vi "Splash Screen Main.vi"() -> ()   [LabVIEW 2020]
uses:
  <vilib>/LAVA/UI Tools/Fading/SetTransparency(U8)__lava_lib_ui_tools.vi
  <vilib>/LAVA/UI Tools/Fading/_Fade In(I32)__lava_lib_ui_tools.vi
  <vilib>/LAVA/UI Tools/Fading/_Fade Out(I32)__lava_lib_ui_tools.vi
panel:
  out "Logo":picture
  out "Status Indicator":string
  out "Splash Indicator Cluster":T1
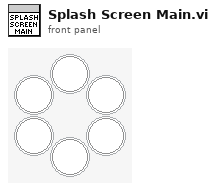
[diagram p1: front panel]
types:
  T1 = cluster{"Indicator 1":bool, "Indicator 2":bool, "Indicator 3":bool, "Indicator 4":bool, "Indicator 5":bool, "Indicator 6":bool}
  T2 = enum32{"Invalid", "Standard", "Closed", "Hidden", "Minimized", "Maximized"}
  T3 = cluster{"Indicator 6":bool, "Indicator 5":bool, "Indicator 3":bool, "Indicator 4":bool, "Indicator 2":bool, "Indicator 1":bool}
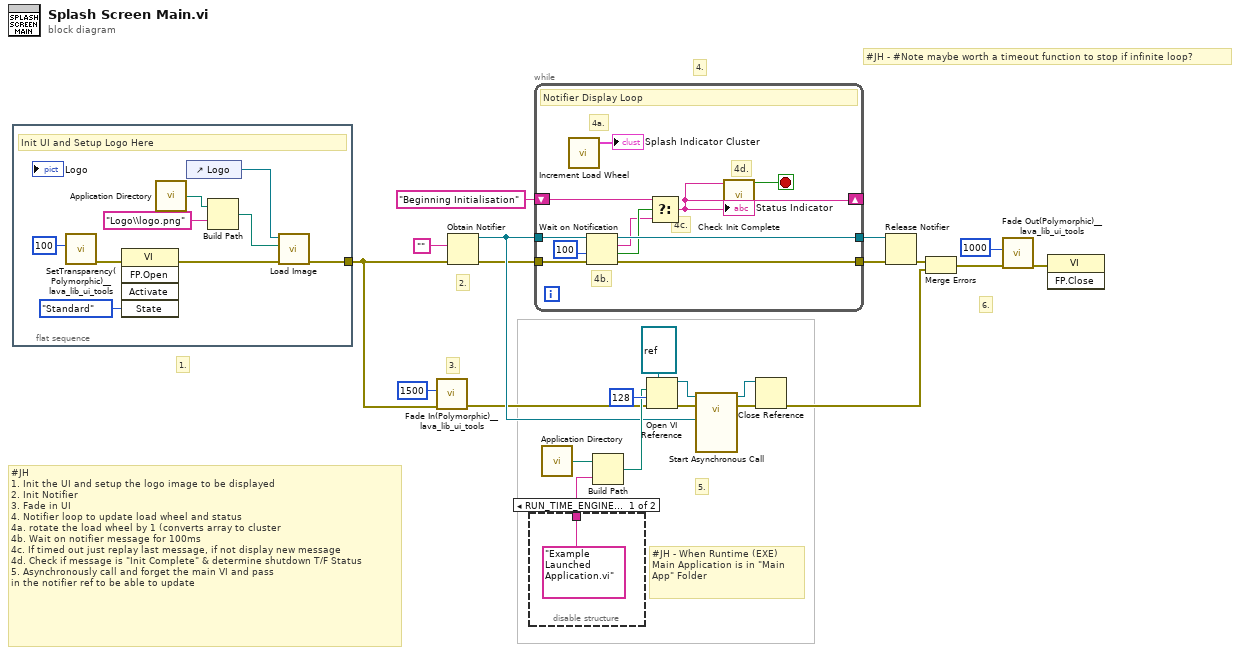
[diagram p0: block diagram]
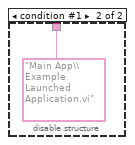
[diagram p2: hidden frame]
diagram:
  # "#JH - When Runtime (EXE)\nMain Application is in \"Main App\" Folder"
  # "#JH - #Note maybe worth a timeout function to stop if infinite loop?"
  # "#JH\n1. Init the UI and setup the logo image to be displayed\n2. Init Notifier\n3. Fade in UI\n4. Notifier loop to update load wheel and status\n4a. rotate the load wheel by 1 (converts array to cluster\n4b. Wait on notifier message for 100ms\n4c. If timed out just replay last message, if not display new message\n4d. Check if message is \"Init Complete\" & determine shutdown T/F Status\n5. Asynchronously call and forget the main VI and pass\nin the notifier ref to be able to update"
  # "6."
  # "5."
  # "4."
  # "3."
  # "2."
  # "1."
  n1 = flat-sequence {
    tunnel: [w31] -> w19
    frame #0 {
      # "Init UI and Setup Logo Here"
      n2 = call-poly <vilib>:"SetTransparency(Polymorphic)__lava_lib_ui_tools.vi"("Transparency (%)"=u8 100) -> ("error out"=w30:errorcluster)  [unwired: 9 in, 1 out]
      n3 = invoke class="VI" method="FP.Open"(error in=w30, "State"=T2."Standard") -> (error out=w27:errorcluster)  [unwired: 3 in, 4 out]
      n4 = call <vilib>:"Application Directory.vi"() -> ("Application Directory"=w26:path)
      n5 = control-ref of="Logo"() -> (w32:refnum<vi>)
      n6 = Build Path(base path=w26, name or relative path="Logo\\logo.png") -> (appended path=w24:path)
      n7 = call "Load Image.vi"("error in (no error)"=w27, "path to PNG file"=w24, "Picture Ref"=w32) -> ("error out"=w31:errorcluster)  [unwired: 8 in]
    }
  }
  n8 = call-poly <vilib>:"Fade In(Polymorphic)__lava_lib_ui_tools.vi"("error in"=w19, "Fade time (ms)"=1500) -> ("error out"=w11:errorcluster)  [unwired: 8 in, 1 out]
  n9 = Obtain Notifier(notification data type="", error in (no error)=w19) -> (notifier out=w12:refnum<notifier>, error out=w7:errorcluster)  [unwired: 2 in, 1 out]
  n10 = disable-structure shown="RUN_TIME_ENGINE==False, Default" {
    disable-tunnel: ["Example Launched Application.vi" "Main App\\Example Launched Application.vi"] -> w14
    frame condition #0 (active) {
    }
    frame condition #1 {
    }
  }
  n11 = while {
    tunnel: w12 -> [w44]
    tunnel: [w43] -> w22
    shift-right: [w38] -> _
    shift-left: "Beginning Initialisation" -> [w40]
    tunnel: w7 -> [w36]
    tunnel: [w35] -> w6
    stop <- w37 stop-if-true
    # "4d."
    # "4c."
    # "4b."
    # "4a."
    # "Notifier Display Loop"
    n12 = call "Increment Load Wheel.vi"() -> ("Splash Indicator Cluster out"=→"Splash Indicator Cluster":T3)  [unwired: 19 in]
    n13 = Wait on Notification(notifier=w44, timeout in ms (-1)=100, error in (no error)=w36) -> (notifier out=w43:refnum<notifier>, notification=w39:string, timed out?=w41:bool, error out=w35:errorcluster)  [unwired: 1 in]
    n14 = Select(t=w40, s=w41, f=w39) -> (s? t:f=w38:string)
    "Status Indicator" <- w38
    n15 = call "Check Init Complete.vi"("String"=w38) -> ("Shutdown (T/F)"=w37:bool)  [unwired: 14 in]
  }
  n16 = call <vilib>:"Application Directory.vi"() -> ("Application Directory"=w1:path)
  n17 = Build Path(base path=w1, name or relative path=w14) -> (appended path=w13:path)
  n18 = Open VI Reference(type specifier VI Refnum (for type only)=refnum<vi> refnum, vi path=w13, options=128, error in (no error)=w11) -> (vi reference=w17:refnum<vi>, error out=w18:errorcluster)  [unwired: 2 in]
  n19 = call-by-ref "Start Asynchronous Call"(reference=w17, error in=w18, "Splash Notifier"=w12) -> (reference out=w9:refnum<vi>, error out=w10:errorcluster)  [unwired: 10 in, 1 out]
  n20 = Close Reference(reference=w9, error in (no error)=w10) -> (error out=w4:errorcluster)
  n21 = Release Notifier(notifier=w22, error in (no error)=w6) -> (error out=w8:errorcluster)  [unwired: 1 in, 2 out]
  n22 = Merge Errors(w8, w4) -> (w5:errorcluster)
  n23 = call-poly <vilib>:"Fade Out(Polymorphic)__lava_lib_ui_tools.vi"("error in"=w5, "Fade time (ms)"=1000) -> ("error out"=w3:errorcluster)  [unwired: 8 in, 1 out]
  n24 = invoke class="VI" method="FP.Close"(error in=w3) -> ()  [unwired: 2 in, 3 out]
